vi "FTW-Test-MessageTransports.vi"() -> (0 "Test Result":errorcluster)   [LabVIEW 2014]
uses:
  src/core/actor/socket/FTW-Socket-MessageTransportScheme.ctl
  src/core/actor/socket/FTW-Socket-Type.ctl
  src/core/error/FTW-ERR-ExceptionType.ctl
  src/core/error/FTW-ERR-Assert-DeveloperError.vi
  src/core/error/FTW-ERR-ThrowError.vi
  src/core/error/FTW-ERR-NoErrorConstant.vi
  src/core/error/FTW-ERR-CallChain.vi
  src/core/string/FTW-STR-ReplaceWhitespace.vi
  src/core/actor/socket/FTW-Socket.lvclass
  src/core/actor/message/FTW-Message.lvclass
  src/core/actor/router/FTW-Router.lvclass
panel:
  in  "Mode":enum32{"Automated Testing", "Manual Control"}(tab)
  in  "Test to Perform":T1(radio)=enum."Parallel: 10x100x10k"
  in  "stop":bool
  out "Results":T3(array[cluster]) {"?" format="%_3p bytes/sec (one-way receive)"; "?" format="%_3f replies/sec"; "?" format="Benchmark Time: %_3psec"}
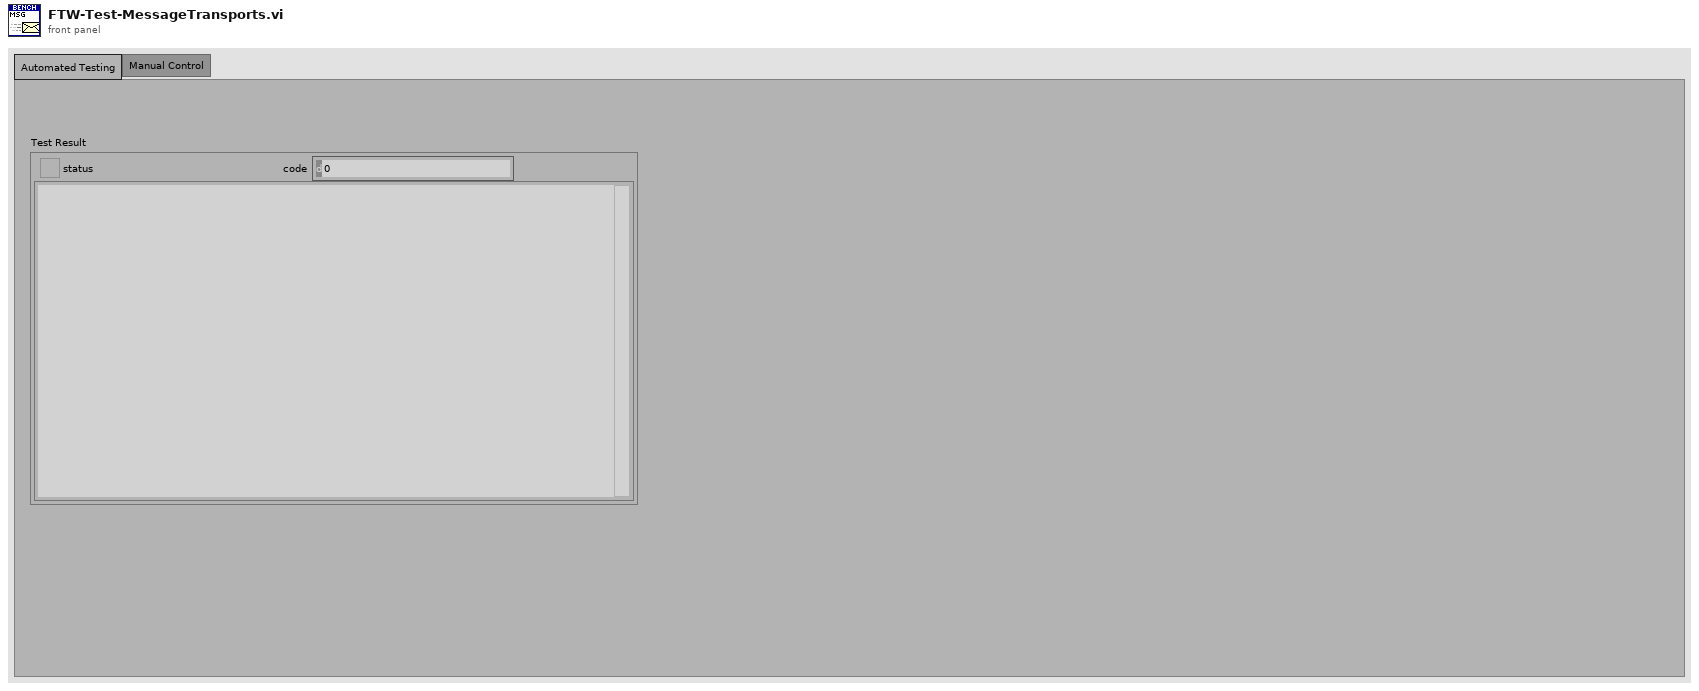
[diagram p1: front panel]
types:
  T1 = enum32{"Serial: 1x1x0", "Serial: 1x1000x0", "Serial: 1x1000x10k", "Serial: 10x100x10k", "Parallel: 10x100x10k", "Parallel: 10x1x10M", "Parallel: 100x1x10k", "Parallel: 100x100x0", "Parallel: 1000x1x1k", "Parallel: 1000x100x10k", "Parallel: 10x100x1M", "Parallel: 1000x1x1M", "Parallel: 10x10000x0"}
  T2 = typedef "FTW-Socket.lvclass/FTW-Socket-MessageTransportScheme.ctl" = enum16{"TCP (tcp://)", "Inter-Process (ipc://)", "In-Process (inproc://)", "WebSocket (ws://)"}
  T3 = cluster{"Server Address":T2, "error":errorcluster, "Client Results":cluster{"Instance":string, "All replies were as expected?":bool}[], dbl, dbl, dbl, "Pass?":bool}[]
  T4 = enum32{"Serial: 1x1x0", "Serial: 1x1000x0", "Serial: 1x1000x10k", "Serial: 10x100x10k", "Parallel: 10x100x10k", "Parallel: 10x1x10M", "Parallel: 100x1x10k", "Parallel: 100x100x0", "Parallel: 1000x1x1k", "Parallel: 1000x100x10k", "Parallel: 10x100x1M", "Parallel: 1000x1x1M", "Parallel: 10x10000x0"}[]
  T5 = cluster{"Inbox Address":T2, "error out":errorcluster, cluster{string, bool}[], "Elapsed Time":dbl, dbl, dbl, bool}[]
  T6 = typedef "FTW-ERR-ExceptionType.ctl" = enum16{"OK", "Info", "Warning", "Error"}
  T7 = typedef "FTW-Socket.lvclass/FTW-Socket-Type.ctl" = enum32{"Server", "Client", "Publisher", "Subscriber", "Pipeline Producer", "Pipeline Consumer", "Surveyor", "Respondent", "Exclusive Pair", "Bus"}
  T8 = cluster{i32, i32, i32, i32, "Replies from Server":i32, "bytes from Server":i32, bool, bool}
  T9 = cluster{"Message Transport Scheme":T2, "error out":errorcluster, cluster{string, bool}[], "Elapsed Time":dbl, dbl, dbl, bool}
  T10 = cluster{"Message Transport Scheme":T2, "error out":errorcluster, cluster{string, bool}[], "Elapsed Time":dbl, dbl, dbl, bool}[]
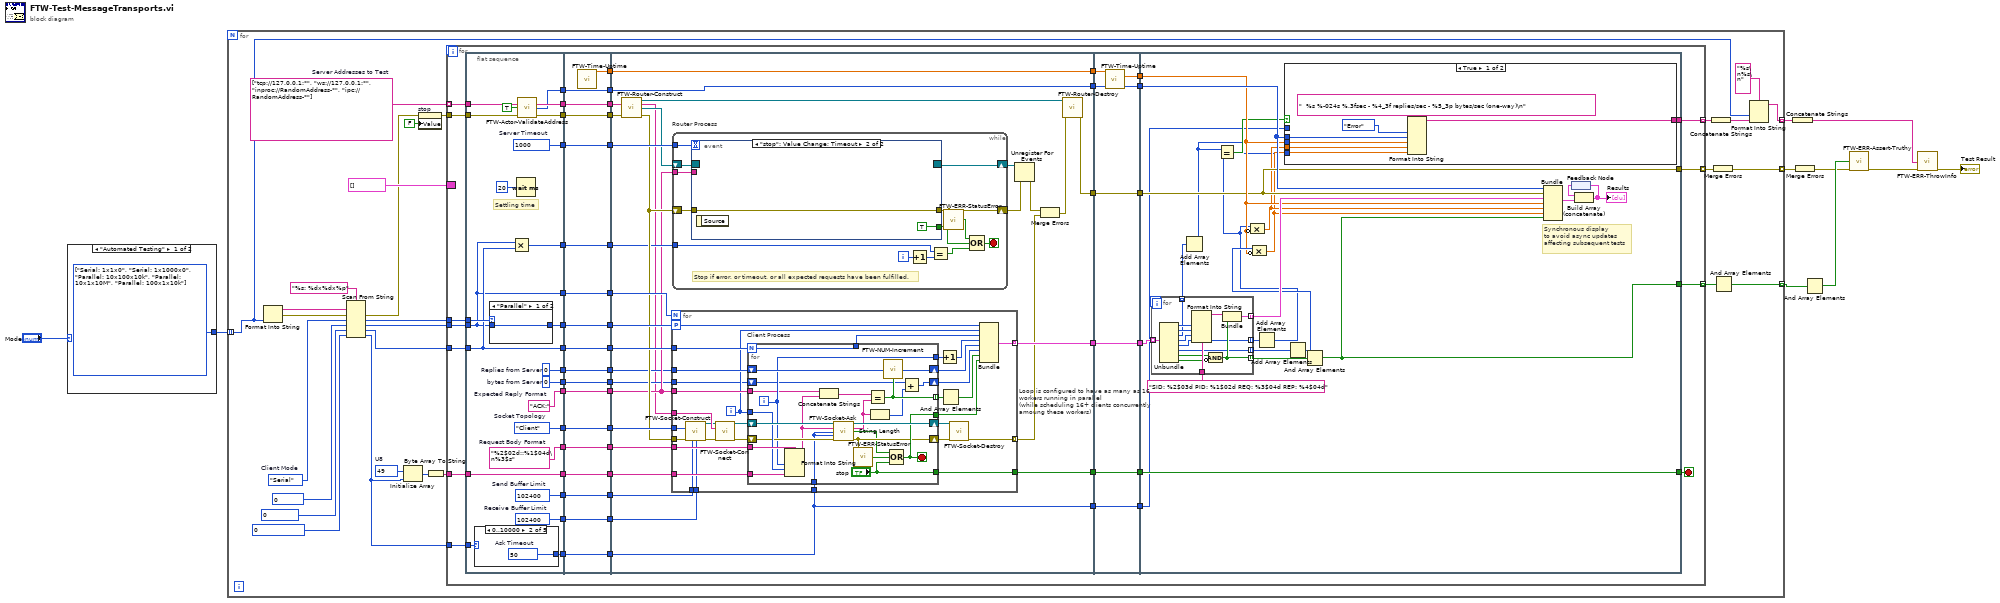
[diagram p0: block diagram]
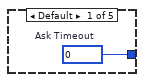
[diagram p2: hidden frame]
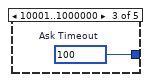
[diagram p3: hidden frame]
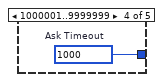
[diagram p4: hidden frame]
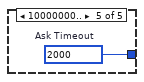
[diagram p5: hidden frame]
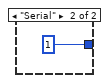
[diagram p6: hidden frame]
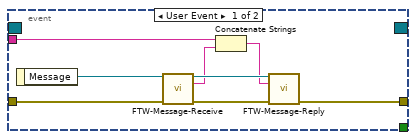
[diagram p7: hidden frame]
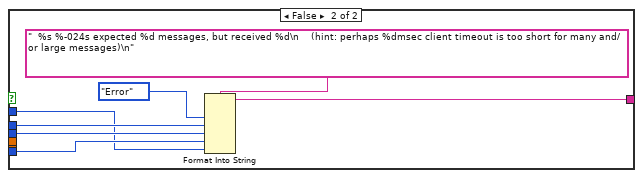
[diagram p8: hidden frame]
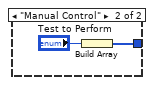
[diagram p9: hidden frame]
diagram:
  n1 = case shown="\"Automated Testing\"" "Mode" {
    tunnel: [w11 w12] -> w9
    frame "Automated Testing" {
      w11 = T4 [enum."Serial: 1x1x0", enum."Serial: 1x1000x0", enum."Parallel: 10x100x10k", enum."Parallel: 10x1x10M", enum."Parallel: 100x1x10k"] items=["Serial: 1x1x0", "Serial: 1x1000x0", "Serial: 1x1000x10k", "Serial: 10x100x10k", "Parallel: 10x100x10k", "Parallel: 10x1x10M", "Parallel: 100x1x10k", "Parallel: 100x100x0", "Parallel: 1000x1x1k", "Parallel: 1000x100x10k", "Parallel: 10x100x1M", "Parallel: 1000x1x1M", "Parallel: 10x10000x0"]
    }
    frame "Manual Control" {
      n2 = Build Array("Test to Perform") -> (w12:T4)
    }
  }
  n3 = for {
    tunnel: w9 -> [w26] mode=indexing
    tunnel: [w32] -> w8 mode=indexing
    tunnel: [w31] -> w7 mode=indexing
    tunnel: [w28] -> w5 mode=indexing
    w23 = enum32{"Parallel", "Serial"}."Serial"  # Client Mode
    w36 = string[] ["tcp://127.0.0.1:*", "ws://127.0.0.1:*", "inproc://RandomAddress-*", "ipc://RandomAddress-*"]  # Server Addresses to Test
    w39 = u8 49  # U8
    n4 = Format Into String(w26) -> (resulting string=w25:string, error out=w24:errorcluster)  [unwired: 3 in]
    n5 = Scan From String(format string="%s: %dx%dx%p", input string=w25, error in=w24, default 1=w23, default 2=0, default 3=0, default 4=0) -> (error out=w21:errorcluster, output 1=w20:enum32{"Parallel", "Serial"}, output 2=w16:i32, output 3=w15:i32, output 4=w14:i32)  [unwired: 1 in, 2 out]
    n6 = Initialize Array(w39, w14) -> (w38:u8[])
    n7 = property on="stop" class="Bool (strict)"(error in=w21, "Value"=FALSE ("stop")) -> (error out=w40:errorcluster)  [unwired: 1 in, 1 out]
    n8 = Byte Array To String(unsigned byte array=w38) -> (string=w37:string)
    n9 = for {
      tunnel: w36 -> [w92] mode=indexing
      tunnel: w16 -> [w89]
      tunnel: w15 -> [w85]
      tunnel: w20 -> [w84]
      tunnel: w40 -> [w83]
      tunnel: w37 -> [w67]
      border: T5 [] -> [_]
      tunnel: [w49] -> w34 mode=indexing
      tunnel: [w48] -> w33 mode=indexing
      tunnel: [w47] -> w30 mode=indexing
      tunnel: w14 -> [w42]
      stop <- w56 stop-if-true
      n10 = flat-sequence {
        tunnel: [w106] -> w99
        tunnel: [w104] -> w93
        tunnel: [w110] -> w90
        tunnel: [w119] -> w86
        tunnel: w83 -> [w107]
        tunnel: w84 -> [w121]
        tunnel: w85 -> [w119]
        tunnel: w89 -> [w110]
        tunnel: w92 -> [w105]
        tunnel: [w112] -> w81
        tunnel: [w101] -> w79
        tunnel: [w120] -> w77
        tunnel: [w118] -> w75
        tunnel: [w113] -> w72
        tunnel: [w116] -> w71
        tunnel: [w117] -> w68
        tunnel: w67 -> [w117]
        tunnel: [w115] -> w65
        tunnel: [w114] -> w59
        tunnel: [w111] -> w58
        tunnel: [w109] -> w52
        tunnel: [w108] -> w50
        tunnel: [w103] -> w45
        tunnel: w42 -> [w100]
        tunnel: [w147] -> w98
        tunnel: [w146] -> w97
        tunnel: w99 -> [w147]
        tunnel: [w145] -> w94
        tunnel: w93 -> [w145]
        tunnel: [w144] -> w91
        tunnel: w90 -> [w144]
        tunnel: [w143] -> w87
        tunnel: w86 -> [w143]
        tunnel: [w142] -> w82
        tunnel: w81 -> [w142]
        tunnel: [w141] -> w80
        tunnel: w79 -> [w141]
        tunnel: [w140] -> w78
        tunnel: w77 -> [w140]
        tunnel: [w139] -> w76
        tunnel: w75 -> [w139]
        tunnel: [w138] -> w74
        tunnel: [w137] -> w73
        tunnel: w72 -> [w137]
        tunnel: w71 -> [w136]
        tunnel: [w136] -> w70
        tunnel: [w135] -> w69
        tunnel: w68 -> [w135]
        tunnel: [w134] -> w66
        tunnel: w65 -> [w134]
        tunnel: w59 -> [w138]
        tunnel: w58 -> [w133]
        tunnel: [w133] -> w57
        tunnel: [w132] -> w53
        tunnel: w52 -> [w132]
        tunnel: [w131] -> w51
        tunnel: w50 -> [w131]
        tunnel: [w130] -> w46
        tunnel: w45 -> [w130]
        tunnel: [w161] -> w96
        tunnel: [w177] -> w95
        tunnel: [w176] -> w88
        tunnel: w76 -> [w159]
        tunnel: w78 -> [w170]
        tunnel: w98 -> [w168]
        tunnel: w97 -> [w177]
        tunnel: w94 -> [w166]
        tunnel: w91 -> [w172]
        tunnel: w87 -> [w173]
        tunnel: w82 -> [w171]
        tunnel: w80 -> [w148]
        tunnel: w74 -> [w157]
        tunnel: w73 -> [w169]
        tunnel: w70 -> [w167]
        tunnel: w69 -> [w160]
        tunnel: w66 -> [w156]
        tunnel: [w150] -> w60
        tunnel: w57 -> [w154]
        tunnel: [w153] -> w54
        tunnel: w53 -> [w152]
        tunnel: w51 -> [w151]
        tunnel: w46 -> [w150]
        tunnel: [w148] -> w43
        tunnel: w96 -> [w262]
        tunnel: w95 -> [w261]
        tunnel: w88 -> [w259]
        tunnel: [w262] -> w64
        tunnel: [w260] -> w63
        tunnel: [w259] -> w62
        tunnel: [w258] -> w61
        tunnel: w60 -> [w258]
        tunnel: [w257] -> w55
        tunnel: w54 -> [w257]
        tunnel: [w256] -> w44
        tunnel: w43 -> [w256]
        tunnel: w64 -> [w270]
        tunnel: w63 -> [w272]
        tunnel: w62 -> [w285]
        tunnel: w61 -> [w274]
        tunnel: [w275] -> w56
        tunnel: w55 -> [w275]
        tunnel: [w273] -> w49
        tunnel: [w271] -> w48
        tunnel: [w270] -> w47
        tunnel: w44 -> [w263]
        frame #0 {
          w108 = 102400  # Receive Buffer Limit
          w109 = 102400  # Send Buffer Limit
          w111 = 0  # bytes from Server
          w112 = 1000  # Server Timeout
          w113 = "%2$02d::%1$04d\n%3$s"  # Request Body Format
          w114 = "ACK:"  # Expected Reply Format
          w115 = 0  # Replies from Server
          w116 = FTW-Socket-Type."Client"  # Socket Topology
          # "Settling time"
          n11 = case shown="0..10000" w100 {
            tunnel: [w123 w124 w125 w126 w127] -> w101
            frame Default {
              w123 = 0  # Ask Timeout
            }
            frame 0..10000 {
              w124 = 50  # Ask Timeout
            }
            frame 10001..1000000 {
              w125 = 100  # Ask Timeout
            }
            frame 1000001..9999999 {
              w126 = 1000  # Ask Timeout
            }
            frame 10000000.. {
              w127 = 2000  # Ask Timeout
            }
          }
          n12 = case shown="\"Parallel\"" w121 {
            tunnel: [w128 1 ("Requests to Send")] -> w120
            tunnel: w110 -> [w128 _]
            frame "Parallel" {
            }
            frame "Serial" {
            }
          }
          n13 = Multiply(x=w110, y=w119) -> (x*y=w118:i32)
          n14 = Wait (ms)(milliseconds to wait=u32 20) -> ()  [unwired: 1 out]
          n15 = call "FTW-Actor-ValidateAddress.vi"("Address"=w105, "Allow wildcard replacement?"=TRUE, "error in"=w107) -> ("Sanitized Address"=w104:string, "Message Transport Scheme"=w103:T2, "error out"=w106:errorcluster)  [unwired: 10 in]
        }
        frame #1 {
          n16 = call "FTW-Time-Uptime.vi"() -> ("Current Uptime"=w146:dbl)  [unwired: 13 in, 2 out]
        }
        frame #2 {
          n17 = call "FTW-Router-Construct.vi"("Inbox Address"=w166, "error in"=w168) -> ("FTW Router"=w165:refnum<class "FTW-Router.lvclass">, "Resolved Inbox Address"=w149:string, "Incoming Message"=w158:refnum<event-registration>, "error out"=w164:errorcluster)  [unwired: 10 in]
          n18 = for "Loop is configured to have as many as 16 workers running in parallel\n(while scheduling 16+ clients concurrently amoung these workers)" {
            N: w172 -> [_]
            tunnel: w164 -> [w196]
            tunnel: w173 -> [w208]
            tunnel: w148 -> [w207]
            workers-P: w170 -> [w204]
            tunnel: [w206] -> w176 mode=indexing
            tunnel: w149 -> [w198]
            tunnel: w157 -> [w203]
            tunnel: w169 -> [w202]
            tunnel: w167 -> [w194]
            tunnel: [w191] -> w155 mode=indexing
            tunnel: w160 -> [w189]
            tunnel: w156 -> [w188]
            tunnel: w154 -> [w183]
            tunnel: [w181] -> w153
            tunnel: w152 -> [w180]
            tunnel: w151 -> [w179]
            i -> [w186]
            n19 = call "FTW-Socket-Construct.vi"("Socket Topology"=w194, "error in"=w196, "Send Buffer Limit"=w180, "Receive Buffer Limit"=w179) -> ("FTW Socket"=w197:refnum<class "FTW-Socket.lvclass">, "error out"=w195:errorcluster)  [unwired: 10 in]
            n20 = call "FTW-Socket-Connect.vi"("FTW Socket"=w197, "Remote Address"=w198, "error in"=w195) -> ("FTW Socket out"=w200:refnum<class "FTW-Socket.lvclass">, "error out"=w199:errorcluster)  [unwired: 11 in]
            n21 = for "Client Process" {
              N: w208 -> [w209]
              shift-right: [w231] -> w193
              shift-left: w200 -> [w232]
              tunnel: w207 -> [w222]
              tunnel: [w227] -> w205
              tunnel: [w221] -> w190 mode=indexing
              tunnel: w203 -> [w214]
              tunnel: w202 -> [w229]
              shift-right: [w224] -> w192
              shift-left: w199 -> [w225]
              tunnel: w186 -> [w228]
              tunnel: w189 -> [w226]
              shift-right: [w220] -> w187
              shift-left: w188 -> [w219]
              tunnel: [w218] -> w185
              shift-right: [w215] -> w182
              shift-left: w183 -> [w211]
              tunnel: ["stop"] -> w181
              tunnel: [w209] -> w178
              i -> [w218]
              stop <- w227 stop-if-true
              n22 = Format Into String(format string=w229, w218, w228, w226) -> (resulting string=w213:string)  [unwired: 2 in, 1 out]
              n23 = Concatenate Strings(w214, w213) -> (w212:string)
              n24 = call "FTW-Socket-Ask.vi"("FTW Socket"=w232, "Request"=w213, "Receive Timeout"=w222, "Send Timeout"=w222, "error in"=w225) -> ("FTW Socket out"=w231:refnum<class "FTW-Socket.lvclass">, "Response"=w217:string, "Timed out?"=w223:bool, "error out"=w224:errorcluster)  [unwired: 6 in, 1 out]
              n25 = call "FTW-ERR-StatusError.vi"("error to check"=w224) -> ("Error?"=w230:bool)
              n26 = Equal?(x=w212, y=w217) -> (x = y?=w221:bool)
              n27 = String Length(string=w217) -> (length=w216:i32)
              n28 = call "FTW-NUM-Increment.vi"("Initial Value"=w219, "Increment?"=w221) -> ("Final Value"=w220:i32)
              n29 = Compound Arithmetic op=OR(w223, w230, "stop") -> (w227:bool)
              n30 = Add(x=w211, y=w216) -> (x+y=w215:i32)
            }
            n31 = Increment(x=w185) -> (x+1=w184:i32)
            n32 = And Array Elements(Boolean array=w190) -> (logical AND=w201:bool)
            n33 = call-dynamic "FTW-Socket-Destroy.vi"("FTW Socket"=w193, "error in"=w192) -> ("error out"=w191:errorcluster)  [unwired: 13 in]
            n34 = Bundle(w204, w186, w178, w184, "Replies from Server"=w187, "bytes from Server"=w182, w201, w205) -> (w206:T8)  [unwired: 1 in]
          }
          n35 = while "Router Process" {
            shift-right: [w244] -> w174
            shift-left: w158 -> [w245]
            shift-right: [w242] -> w175
            shift-left: w164 -> [w243]
            tunnel: w159 -> [w237]
            tunnel: w171 -> [w236]
            tunnel: w157 -> [w233]
            i -> [w235]
            stop <- w238 stop-if-true
            # "Stop if error, or timeout, or all expected requests have been fulfilled."
            n36 = event shown="[1] \"stop\": Value Change;  Timeout" {
              selector: w245 -> [_ _]
              dyn-events: [_ _] -> w244
              timeout: w236 -> [_ _]
              tunnel: [_ TRUE] -> w240
              tunnel: w243 -> [w253 w254]
              tunnel: [w251 w254] -> w242
              tunnel: w233 -> [w249 _]
              event User Event {
                n37 = event-data() -> ("Message"=w252:refnum<class "FTW-Message.lvclass">)  [unwired: 1 in]
                n38 = call "FTW-Message-Receive.vi"("FTW Incoming Message"=w252, "error in"=w253) -> ("FTW Incoming Message out"=w250:refnum<class "FTW-Message.lvclass">, "Message"=w248:string, "error out"=w247:errorcluster)  [unwired: 11 in]
                n39 = Concatenate Strings(w249, w248) -> (w246:string)
                n40 = call "FTW-Message-Reply.vi"("FTW Incoming Message"=w250, "Response"=w246, "error in"=w247) -> ("error out"=w251:errorcluster)  [unwired: 11 in, 1 out]
              }
              event "stop": Value Change; Timeout {
                n41 = event-data() -> ()  [unwired: 1 in, 1 out]
              }
            }
            n42 = Increment(x=w235) -> (x+1=w234:i32)
            n43 = Equal?(x=w237, y=w234) -> (x = y?=w239:bool)
            n44 = call "FTW-ERR-StatusError.vi"("error to check"=w242) -> ("Error?"=w241:bool)
            n45 = Compound Arithmetic op=OR(w241, w240, w239) -> (w238:bool)
          }
          n46 = Unregister For Events(event registration refnum=w174, error in=w175) -> (error out=w163:errorcluster)
          n47 = Merge Errors(w163, w155) -> (w162:errorcluster)
          n48 = call "FTW-Router-Destroy.vi"("FTW Router"=w165, "error in"=w162) -> ("error out"=w161:errorcluster)  [unwired: 13 in]
        }
        frame #3 {
          n49 = call "FTW-Time-Uptime.vi"("Previous Uptime"=w261) -> ("Elapsed Time"=w260:dbl)  [unwired: 12 in, 2 out]
        }
        frame #4 {
          # "Synchronous display\nto avoid async updates\naffecting subsequent tests"
          n50 = for {
            tunnel: w285 -> [w312] mode=indexing
            tunnel: "SID: %2$03d PID: %1$02d REQ: %3$04d REP: %4$04d" -> [w311]
            tunnel: [w307] -> w282 mode=indexing
            tunnel: [w306] -> w284 mode=indexing
            tunnel: [w303] -> w280 mode=indexing
            tunnel: [w302] -> w276 mode=indexing
            tunnel: [w300] -> w267 mode=indexing
            n51 = Unbundle(w312) -> (w310:i32, w309:i32, w300:i32, w301:i32, "Replies from Server"=w302:i32, "bytes from Server"=w303:i32, w304:bool, w305:bool)
            n52 = Format Into String(format string=w311, w310, w309, w301, w302) -> (resulting string=w308:string)  [unwired: 2 in, 1 out]
            n53 = Compound Arithmetic op=AND(w304, invert w305) -> (w306:bool)
            n54 = Bundle(w308, w306) -> (w307:cluster{string, bool})  [unwired: 1 in]
          }
          n55 = Add Array Elements(numeric array=w267) -> (sum=w265:i32)
          n56 = Add Array Elements(numeric array=w276) -> (sum=w264:i32)
          n57 = Equal?(x=w265, y=w264) -> (x = y?=w266:bool)
          n58 = Compound Arithmetic op=MULTIPLY(w264, invert w272) -> (w269:dbl)
          n59 = Add Array Elements(numeric array=w280) -> (sum=w277:i32)
          n60 = Compound Arithmetic op=MULTIPLY(w277, invert w272) -> (w268:dbl)
          n61 = case shown="True" w266 {
            tunnel: w274 -> [w292 w299]
            tunnel: [w290 w297] -> w273
            tunnel: w272 -> [w289 _]
            tunnel: w269 -> [w288 _]
            tunnel: w268 -> [w287 _]
            tunnel: w265 -> [_ w296]
            tunnel: w264 -> [_ w295]
            tunnel: w263 -> [_ w294]
            frame True {
              n62 = Format Into String(format string="  %s %-024s %.3fsec - %4_3f replies/sec - %5_3p bytes/sec (one-way)\n", FTW-ERR-ExceptionType."Error" ("Exception"), w292, w289, w288, w287) -> (resulting string=w290:string)  [unwired: 2 in, 1 out]
            }
            frame False {
              n63 = Format Into String(format string="  %s %-024s expected %d messages, but received %d\n    (hint: perhaps %dmsec client timeout is too short for many and/or large messages)\n", FTW-ERR-ExceptionType."Error" ("Exception"), w299, w296, w295, w294) -> (resulting string=w297:string)  [unwired: 2 in, 1 out]
            }
          }
          n64 = And Array Elements(Boolean array=w284) -> (logical AND=w271:bool)
          n65 = Bundle("Message Transport Scheme"=w274, "error out"=w270, w282, "Elapsed Time"=w272, w269, w268, w271) -> (w279:T9)  [unwired: 1 in]
          n66 = feedback #1() -> (w283:T5)
          n67 = Build Array (concatenate)(w283, w279) -> (w278:T10)
          "Results" <- w278
          n68 = feedback-in #1(w278) -> ()
        }
      }
    }
    n69 = Concatenate Strings(w34) -> (w29:string)
    n70 = Merge Errors(w30) -> (w31:errorcluster)
    n71 = And Array Elements(Boolean array=w33) -> (logical AND=w32:bool)
    n72 = Format Into String(format string="%s\n%s\n", w26, w29) -> (resulting string=w28:string)  [unwired: 2 in, 1 out]
  }
  n73 = Concatenate Strings(w5) -> (w4:string)
  n74 = Merge Errors(w7) -> (w2:errorcluster)
  n75 = And Array Elements(Boolean array=w8) -> (logical AND=w3:bool)
  n76 = call "FTW-ERR-Assert-Truthy.vi"("Expected Truthy"=w3, "error in"=w2) -> ("error out"=w1:errorcluster)  [unwired: 13 in]
  n77 = call "FTW-ERR-ThrowInfo.vi"("Informational Message"=w4, "error in"=w1) -> ("error out"=→"Test Result":errorcluster)  [unwired: 13 in]
